vi "Example_Sweep.vi"() -> ()   [LabVIEW 2019]
uses:
  Instrument.DAQ/Typedefs/AO.Channel--Cluster--Array.ctl
  Instrument.DAQ/Typedefs/AO.Channel--Cluster.ctl
  Instrument.DAQ/Typedefs/AO.Channel.Function--Enum.ctl
  Instrument.DAQ/Typedefs/Sweep.Configuration--Cluster.ctl
  Instrument.DAQ/Typedefs/Sweep.Channel--Cluster--Array.ctl
  Instrument.DAQ/Typedefs/Sweep.Channel--Cluster.ctl
  Instrument.DAQ/Typedefs/Sweep.Pattern--Enum.ctl
  Instrument.DAQ/Typedefs/REF.Channel--Cluster--Array.ctl
  Instrument.DAQ/Typedefs/REF.Channel--Cluster.ctl
  Instrument.Lockin/Instrument.Lockin.lvclass
  Instrument.DAQ/Instrument.DAQ.lvclass
panel:
  in  "Channels: Lockin":T1=[{"Enable?"=TRUE, "Channel"=1, "Frequency"=20.0, "Phase"=0.0, "TC"=0.1, "Roll-Off"=2}] {"Roll-Off" min=1; "TC" min=0.0001 format="%#_3p"; "Phase" format="%#_3g"; "Frequency" min=0.0001 max=200000.0 format="%#_6p"; "Channel" min=1}
  in  "Configure Sweep":T3={"Sweep Time (s)"=10.0, "Initial Wait (s)"=1.0, "Return to Start"=FALSE, "Channels"=[{"Enable?"=FALSE, "Channel"=5, "Start"=0.0, "End"=0.1, "Pattern"=enum."Ramp /", "Table"=[]}]} {"Channels"."Table" format="%#_1f"; "Channels"."Channel" min=1 max=128; "Channels"."Start" format="%#_6p"; "Channels"."End" format="%#_6p"; "Initial Wait (s)" format="%#_6p"}
  out "2 terminal":cluster{"Y":dbl[], "Y":dbl[]}(graph)
  out "4 terminal":cluster{"Y":dbl[], "Y":dbl[]}(graph)
  in  "Channels: AO":T7=[{"Enable?"=TRUE, "Channel"=1, "Amplitude"=0.05, "Offset"=0.0, "Frequency"=20.0, "Phase"=0.0, "Function"=enum."sine", "Sweeping?"=FALSE, "Limit AC"=FALSE, "Limit DC?"=FALSE, "Duty Cycle"=FALSE}, {"Enable?"=TRUE, "Channel"=2, "Amplitude"=0.0, "Offset"=0.0, "Frequency"=0.1, "Phase"=0.0, "Function"=enum."sine", "Sweeping?"=FALSE, "Limit AC"=FALSE, "Limit DC?"=FALSE, "Duty Cycle"=FALSE}, {"Enable?"=TRUE, "Channel"=3, "Amplitude"=0.0, "Offset"=0.0, "Frequency"=0.1, "Phase"=0.0, "Function"=enum."sine", "Sweeping?"=FALSE, "Limit AC"=FALSE, "Limit DC?"=FALSE, "Duty Cycle"=FALSE}, {"Enable?"=TRUE, "Channel"=4, "Amplitude"=0.0, "Offset"=0.0, "Frequency"=0.1, "Phase"=0.0, "Function"=enum."sine", "Sweeping?"=FALSE, "Limit AC"=FALSE, "Limit DC?"=FALSE, "Duty Cycle"=FALSE}, {"Enable?"=TRUE, "Channel"=5, "Amplitude"=0.0, "Offset"=0.0, "Frequency"=0.1, "Phase"=0.0, "Function"=enum."sine", "Sweeping?"=FALSE, "Limit AC"=FALSE, "Limit DC?"=FALSE, "Duty Cycle"=FALSE}] {"Phase" format="%#_3g"; "Frequency" min=0.0001 max=200000.0 format="%#_6p"; "Offset" format="%#_6p"; "Amplitude" min=0.0 max=10.0 format="%#_6p"}
  # "Lockin Example: Sweep\nMake Sure Lockin Program is running!"
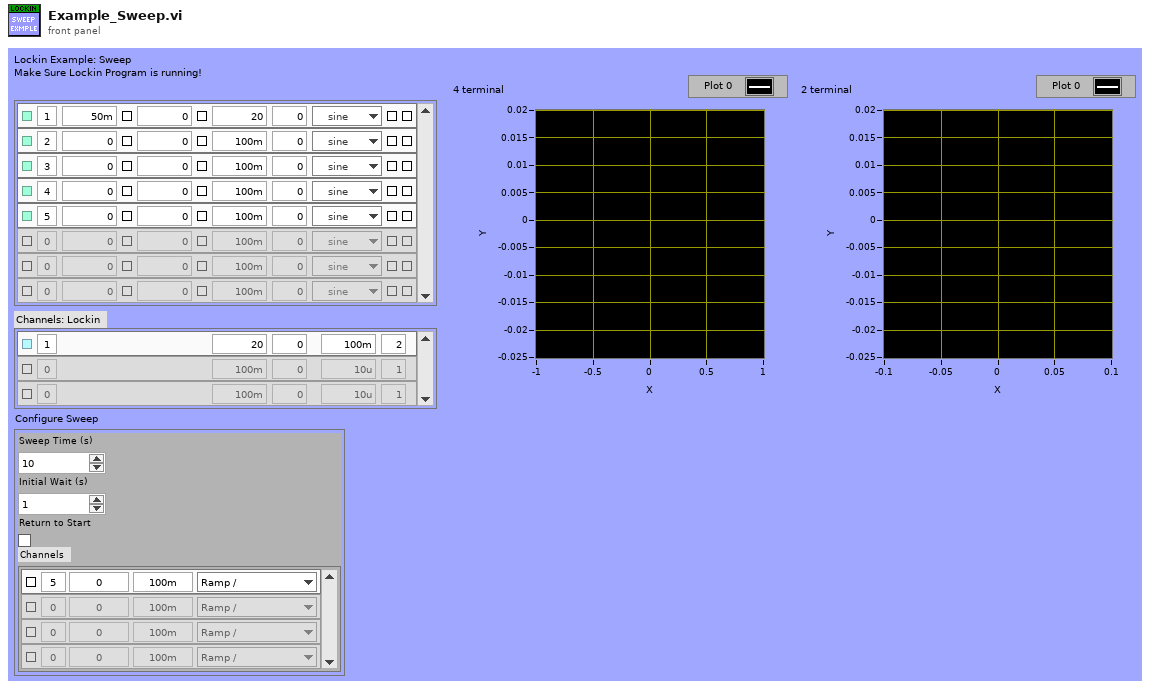
[diagram p1: front panel]
types:
  T1 = typedef "Instrument.Lockin.lvlib/Instrument.DAQ.lvclass/REF.Channel--Cluster--Array.ctl" = T2[]
  T2 = typedef "Instrument.Lockin.lvlib/Instrument.DAQ.lvclass/REF.Channel--Cluster.ctl" = cluster{"Enable?":bool, "Channel":i32, "Frequency":dbl, "Phase":dbl, "TC":dbl, "Roll-Off":i32}
  T3 = typedef "Instrument.Lockin.lvlib/Instrument.DAQ.lvclass/Sweep.Configuration--Cluster.ctl" = cluster{"Sweep Time (s)":dbl, "Initial Wait (s)":dbl, "Return to Start":bool, "Channels":T4}
  T4 = typedef "Instrument.Lockin.lvlib/Instrument.DAQ.lvclass/Sweep.Channel--Cluster--Array.ctl" = T5[]
  T5 = typedef "Instrument.Lockin.lvlib/Instrument.DAQ.lvclass/Sweep.Channel--Cluster.ctl" = cluster{"Enable?":bool, "Channel":u16, "Start":dbl, "End":dbl, "Pattern":T6, "Table":dbl[]}
  T6 = typedef "Instrument.Lockin.lvlib/Instrument.DAQ.lvclass/Sweep.Pattern--Enum.ctl" = enum16{"Ramp /", "Ramp /\\", "Smooth Ramp _/", "Smooth Ramp _/\\_", "Table"}
  T7 = typedef "Instrument.Lockin.lvlib/Instrument.DAQ.lvclass/AO.Channel--Cluster--Array.ctl" = T8[]
  T8 = typedef "Instrument.Lockin.lvlib/Instrument.DAQ.lvclass/AO.Channel--Cluster.ctl" = cluster{"Enable?":bool, "Channel":i32, "Amplitude":dbl, "Offset":dbl, "Frequency":dbl, "Phase":dbl, "Function":T9, "Sweeping?":bool, "Limit AC":bool, "Limit DC?":bool, "Duty Cycle":bool}
  T9 = typedef "Instrument.Lockin.lvlib/Instrument.DAQ.lvclass/AO.Channel.Function--Enum.ctl" = enum16{"sine", "square", "triangle", "saw"}
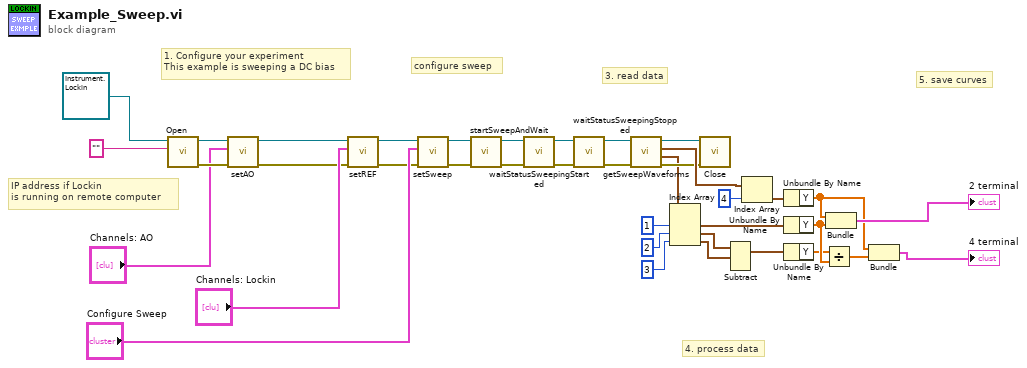
[diagram p0: block diagram]
diagram:
  # "5. save curves"
  # "4. process data"
  # "3. read data"
  # "1. Configure your experiment\nThis example is sweeping a DC bias"
  # "configure sweep"
  # "IP address if Lockin\nis running on remote computer"
  n1 = call-dynamic "Open.vi"("address"="", "Instrument.Lockin in"=refnum<class "Instrument.Lockin.lvclass"> refnum) -> ("error out"=w36:errorcluster, "Instrument.Lockin out"=w38:refnum<class "Instrument.Lockin.lvclass">)  [unwired: 8 in]
  n2 = call-dynamic "setAO.vi"("error in (no error)"=w36, "Channels: AO"="Channels: AO", "Instrument.Lockin in"=w38) -> ("error out"=w22:errorcluster, "Instrument.Lockin out"=w21:refnum<class "Instrument.Lockin.lvclass">)  [unwired: 7 in]
  n3 = call-dynamic "setREF.vi"("error in (no error)"=w22, "Channels: Lockin in"="Channels: Lockin", "Instrument.Lockin in"=w21) -> ("error out"=w19:errorcluster, "Instrument.Lockin out"=w20:refnum<class "Instrument.Lockin.lvclass">)  [unwired: 7 in]
  n4 = call-dynamic "setSweep.vi"("error in (no error)"=w19, "Configure Sweep"="Configure Sweep", "Instrument.Lockin in"=w20) -> ("error out"=w27:errorcluster, "Instrument.Lockin out"=w28:refnum<class "Instrument.Lockin.lvclass">)  [unwired: 7 in]
  n5 = call-dynamic "startSweepAndWait.vi"("error in (no error)"=w27, "Instrument.Lockin in"=w28) -> ("error out"=w18:errorcluster, "Instrument.Lockin out"=w17:refnum<class "Instrument.Lockin.lvclass">)  [unwired: 8 in]
  n6 = call-dynamic "waitStatusSweepingStarted.vi"("error in (no error)"=w18, "Instrument.Lockin in"=w17) -> ("error out"=w15:errorcluster, "Instrument.Lockin out"=w16:refnum<class "Instrument.Lockin.lvclass">)  [unwired: 8 in]
  n7 = call-dynamic "waitStatusSweepingStopped.vi"("error in (no error)"=w15, "Instrument.Lockin in"=w16) -> ("error out"=w14:errorcluster, "Instrument.Lockin out"=w13:refnum<class "Instrument.Lockin.lvclass">)  [unwired: 8 in]
  n8 = call-dynamic "getSweepWaveforms.vi"("error in (no error)"=w14, "Instrument.Lockin in"=w13) -> ("error out"=w24:errorcluster, "Sweep_AI"=w12:waveform(dbl)[], "Sweep_AO"=w29:waveform(dbl)[], "Instrument.Lockin out"=w25:refnum<class "Instrument.Lockin.lvclass">)  [unwired: 6 in]
  n9 = Index Array(array=w12, index #1=1 ("index"), index #2=2 ("index"), index #3=3 ("index")) -> (element #1=w33:waveform(dbl), element #2=w8:waveform(dbl), element #3=w6:waveform(dbl))
  n10 = call-dynamic "Close.vi"("error in (no error)"=w24, "Instrument.Lockin in"=w25) -> ()  [unwired: 8 in, 2 out]
  n11 = Subtract(1:w6, 2:w8) -> (0:w7:waveform(dbl))  [unwired: 1 in, 1 out]
  n12 = Index Array(array=w29, index=4) -> (element=w32:waveform(dbl))
  n13 = Unbundle By Name(w32) -> ("Y"=w1:dbl[])
  n14 = Unbundle By Name(w33) -> ("Y"=w4:dbl[])
  n15 = Unbundle By Name(w7) -> ("Y"=w3:dbl[])
  n16 = Divide(x=w3, y=w4) -> (x/y=w2:dbl[])
  n17 = Bundle("Y"=w1, "Y"=w4) -> (→"2 terminal":cluster{"Y":dbl[], "Y":dbl[]})  [unwired: 1 in]
  n18 = Bundle("Y"=w1, w2) -> (→"4 terminal":cluster{"Y":dbl[], dbl[]})  [unwired: 1 in]
